vi "Variant to JSON Text.vi"(4 "LVClass Serializer":refnum<class "JSONtext LVClass Serializer.lvclass">, 5 "enable LabVIEW extensions? (T)":bool=TRUE, 6 "Pretty Print?":bool, 8 "error in (no error)":errorcluster, 10 "Variant":variant) -> (0 "error out":errorcluster, 1 "Name of data in Variant":string, 3 "<JSON>":string)   [LabVIEW 2020, in "JSONtext.lvlib"]
doc: "Converts a LabVIEW datatype (<b>Variant</b>) into a JSON value. \n\nStrings or Arrays of strings marked with a leading \"<JSON>\" tag in their name (including inside clusters) are treated as already being valid JSON. Strings not marked as <JSON> are quoted and escaped as a JSON String. Note that JSONtext.lvlib functions that produce JSON have their outputs labelled \"<JSON>\", so that they may be used as inputs to other functions.\n\nTwo types of LabVIEW Clusters are supported: either with all named elements, which are converted to JSON Objects, or all unnamed elements (or elements just named \"<JSON>\"), which are converted to a JSON Array. Handling of mixed clusters with some named and some unnamed in undefined (currently, this VI will use the first element to determine whether to convert to an Object or Array)."
uses:
  <vilib>/JDP Science/JSONtext/JSONtext.lvlib
  <vilib>/JDP Science/JSONtext/LVClass Serializer/JSONtext LVClass Serializer.lvclass
  <vilib>/Utility/Data Type/Type Definitions/Data Type.ctl
  <vilib>/JDP Science/JSONtext/support/Remove trailing zeros.vi
  <vilib>/JDP Science/JSONtext/support/quote and escape json string 2.vi
  <vilib>/JDP Science/JSONtext/Base64/base64url Encode.vi
  <vilib>/JDP Science/JSONtext/support/Format JSON Object.vi
  <vilib>/Utility/Data Type/NI_Data Type.lvlib
  <vilib>/JDP Science/JDP Science Common Utilities/JDP Utility.lvlib
  <vilib>/JDP Science/JDP Science Common Utilities/Timestamp/JDP Timestamp.lvlib
  <vilib>/JDP Science/JSONtext/support/Set Map/SetMap.lvlib
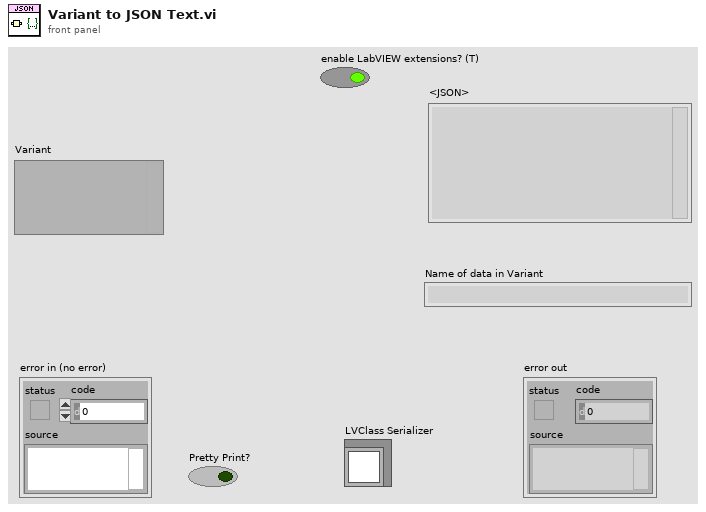
[diagram p1: front panel]
types:
  T1 = typedef "NI_Data Type.lvlib/Data Type.ctl" = enum8{"Invalid Type", "Void", "I8", "I16", "I32", "I64", "U8", "U16", "U32", "U64", "Single Float", "Double Float", "Extended Float", "Single Complex", "Double Complex", "Extended Complex", "Enum U8", "Enum U16", "Enum U32", "Enum U64", "Single Float With Unit", "Double Float With Unit", "Extended Float With Unit", "Single Complex with Unit", "Double Complex with Unit", "Extended Complex with Unit", "Boolean", "String", "Path", "Picture", "Tag", "Array", "Cluster", "Variant", "LV Variant", "Waveform", "Timestamp", "Digital Waveform", "Digital Data", "ExpressData", "Refnum", "External Data", "VI", "Poly VI", "LabVIEW Class Instance", "Fixed Point", "Set Collection", "Map Collection"}
  T2 = typedef "JSONtext.lvlib/Tag Type.ctl" = enum16{"No Tag", "<JSON>", "<JOBJ>"}
  T3 = cluster{"<JSON>attributes":string, "t0":timestamp, "dt":dbl, "Y":dbl[]}
  T4 = typedef "NI_Data Type.lvlib/Refnum Type.ctl" = enum16{"NotARefnum", "UnknownRefnum", "Generic", "Datalog", "ByteStream", "Device", "Occurence", "TCPNetConnection", "Auto", "Menu", "Imaq", "Hardware", "DataSocket", "Visa", "IVI", "UDPNetConnection", "Notifier", "Queue", "Irda", "EventReg", "DotNet", "UserEvent", "Callback", "UNUSED_EMPTY_POSITION", "BlueToothNetConnection", "LVObjApp", "LVObjVI", "LVObjUnknown", "GenericClass", "UserDefinedRefnumTag", "DataValue", "RT FIFO", "TDMS File", "PythonSessionRefnum"}
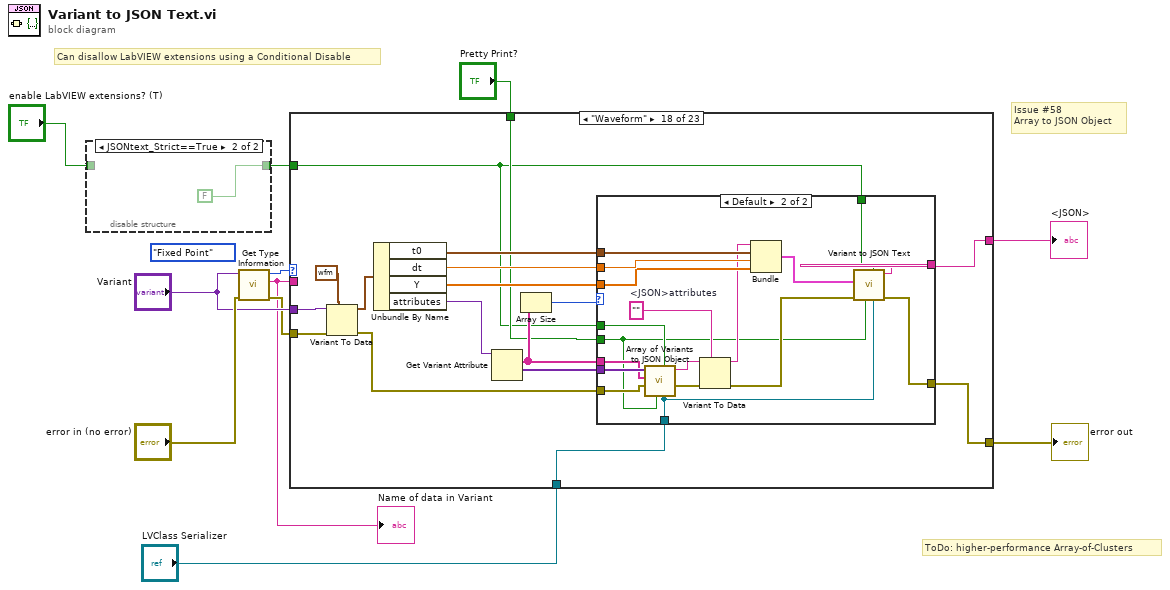
[diagram p0: block diagram]
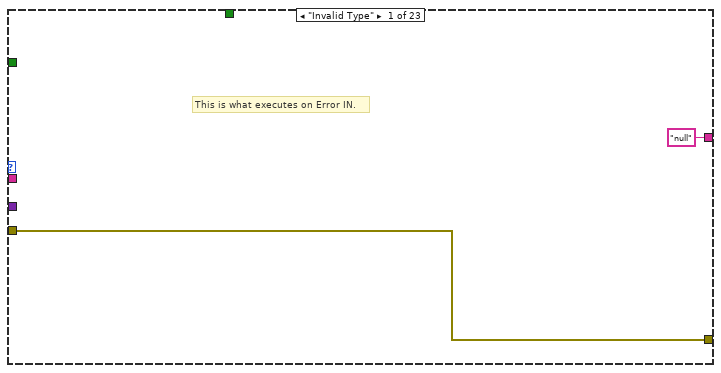
[diagram p3: hidden frame]
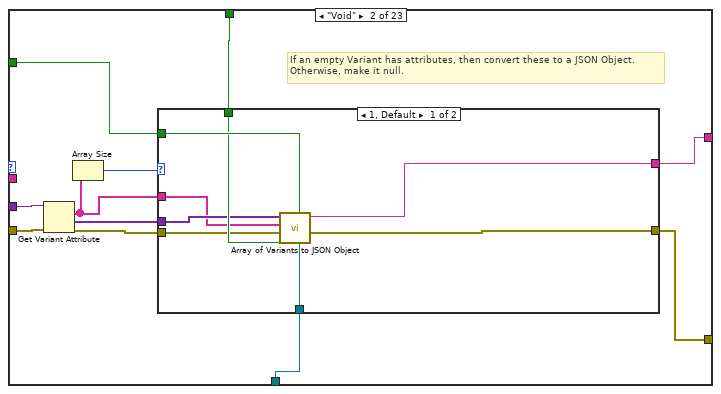
[diagram p4: hidden frame]
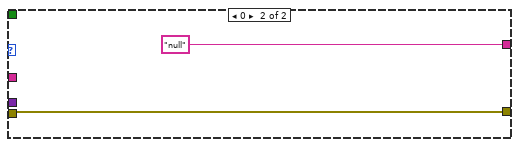
[diagram p5: hidden frame]
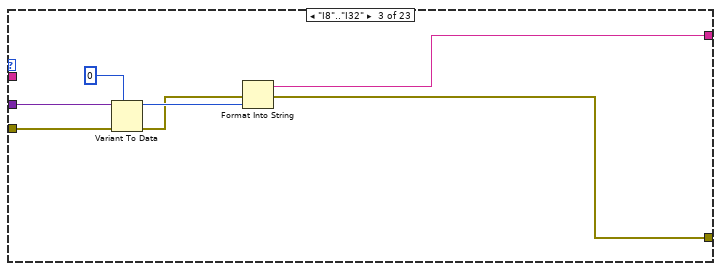
[diagram p6: hidden frame]
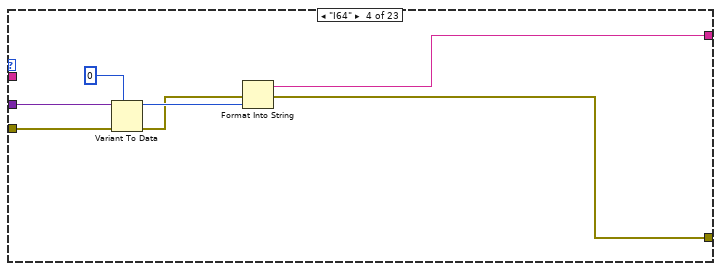
[diagram p7: hidden frame]
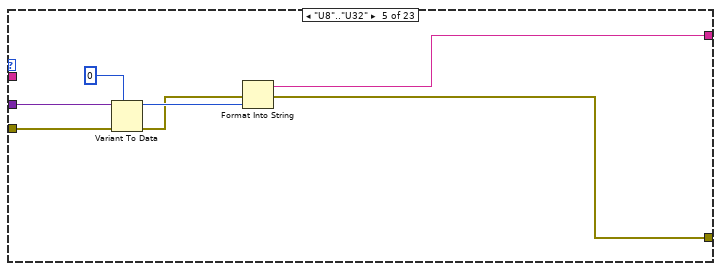
[diagram p8: hidden frame]
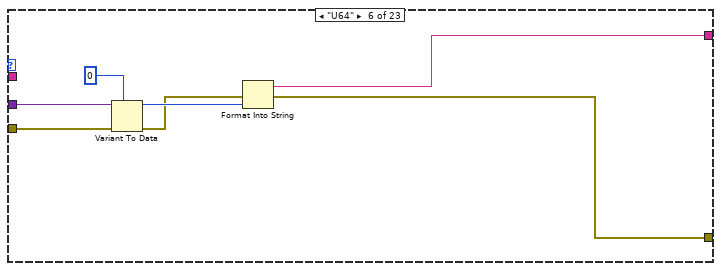
[diagram p9: hidden frame]
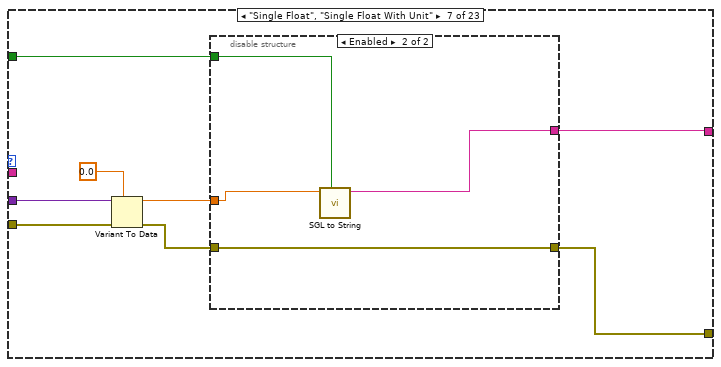
[diagram p10: hidden frame]
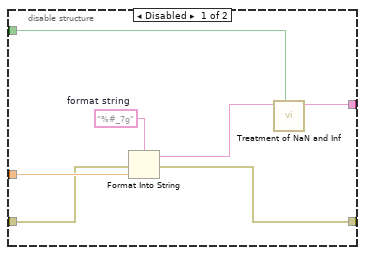
[diagram p11: hidden frame]
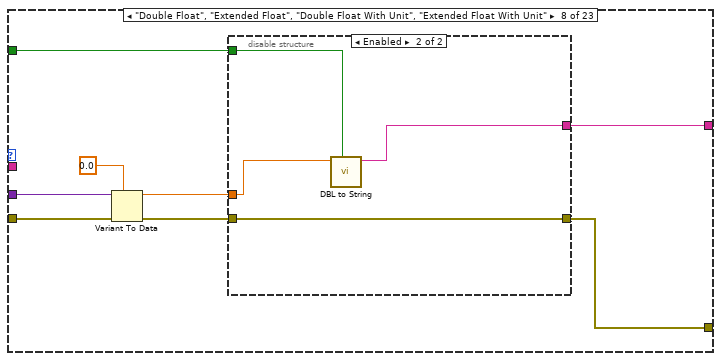
[diagram p12: hidden frame]
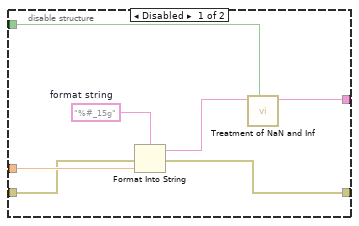
[diagram p13: hidden frame]
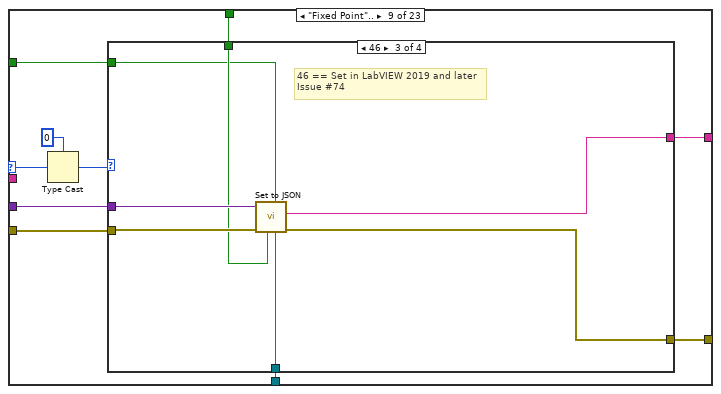
[diagram p14: hidden frame]
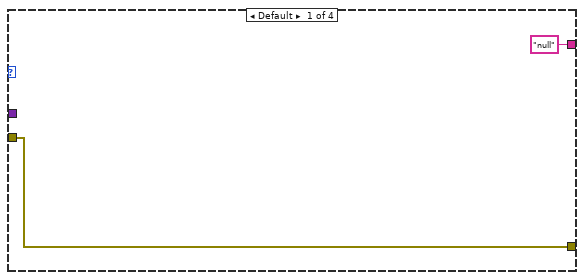
[diagram p15: hidden frame]
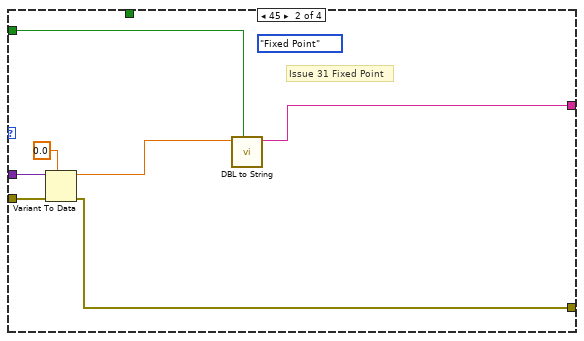
[diagram p16: hidden frame]
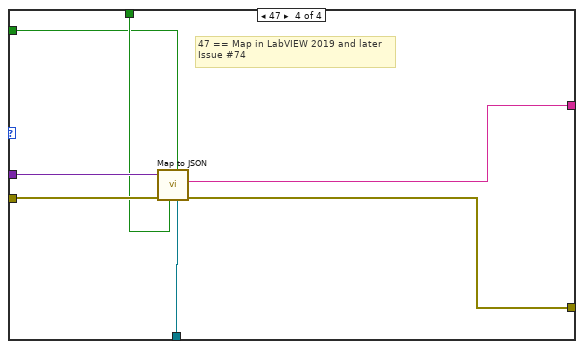
[diagram p17: hidden frame]
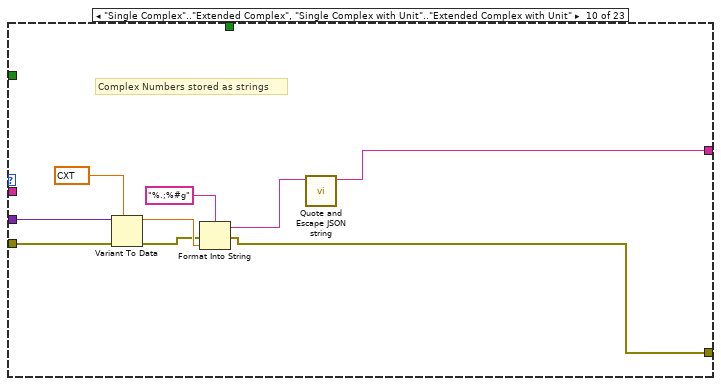
[diagram p18: hidden frame]
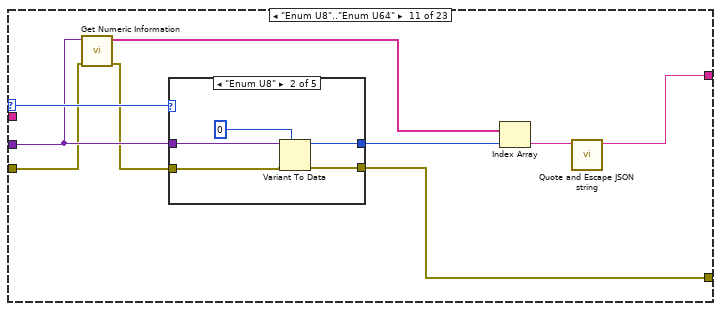
[diagram p19: hidden frame]
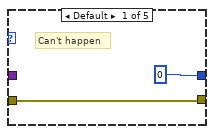
[diagram p20: hidden frame]
diagram:
  (unwired) Data_Type."Fixed Point" ("Type")
  # "ToDo: higher-performance Array-of-Clusters"
  # "Issue #58\nArray to JSON Object"
  # "Can disallow LabVIEW extensions using a Conditional Disable"
  n1 = disable-structure shown="JSONtext_Strict==True" {
    disable-tunnel: "enable LabVIEW extensions? (T)" -> [w12 _]
    disable-tunnel: [w12 FALSE ("enable LabVIEW extensions? (T)")] -> w3
    frame condition #0 (active) {
    }
    frame condition #1 {
    }
  }
  n2 = call <vilib>:"Get Type Information.vi"("error in (no error)"="error in (no error)", "variant"="Variant") -> ("error out"=w6:errorcluster, "name"=w4:string, "type"=w5:T1)  [unwired: 5 in, 2 out]
  "Name of data in Variant" <- w4
  n3 = case shown="\"Waveform\"" w5 {
    selector: w5 -> [_ _ _ _ _ _ _ _ w107 _ w152 _ _ _ _ _ _ _ _ _ _ _ _]
    tunnel: "Variant" -> [_ w25 w43 w50 w57 w64 w72 w91 w112 w144 w148 w183 w192 w204 w217 w713 w733 w754 w789 w794 w818 w830 w845]
    tunnel: [w14 w26 w37 w44 w51 w58 w67 w86 w110 w136 w147 w176 w188 w198 w218 w708 w737 w741 w783 w792 w816 w824 w842] -> w10
    tunnel: w6 -> [w14 w20 w41 w48 w55 w62 w70 w89 w111 w143 w146 w181 w187 w202 w216 w711 w732 w753 w787 w793 w817 w829 w842]
    tunnel: w4 -> [_ _ _ _ _ _ _ _ _ _ _ _ w185 _ w208 _ _ _ _ _ _ _ _]
    tunnel: ["null" ("<JSON>") w19 w39 w46 w53 w60 w66 w85 w109 w137 w150 w177 w186 w199 w210 w709 w729 w743 w784 w791 w815 w826 w843] -> w8
    tunnel: "Pretty Print?" -> [_ w18 _ _ _ _ _ _ w104 _ _ _ _ _ w211 w707 w731 w740 _ _ _ w819 _]
    tunnel: w3 -> [_ w17 _ _ _ _ w65 w84 w108 _ _ _ _ _ w209 w703 w730 w739 _ _ _ w820 _]
    tunnel: "LVClass Serializer" -> [_ w16 _ _ _ _ _ _ w103 _ _ _ _ _ w205 w702 w728 w738 _ _ _ w821 _]
    frame "Invalid Type" {
      # "This is what executes on Error IN."
    }
    frame "Void" {
      # "If an empty Variant has attributes, then convert these to a JSON Object.\nOtherwise, make it null."
      n4 = Get Variant Attribute(Variant=w25, error in=w20) -> (names=w23:string[], values=w22:variant[], error out=w21:errorcluster)  [unwired: 2 in, 1 out]
      n5 = Array Size(array=w23) -> (size(s)=w24:i32)
      n6 = case shown="1, Default" w24 {
        tunnel: [w28 w35] -> w26
        tunnel: w23 -> [w30 _]
        tunnel: w22 -> [w31 _]
        tunnel: w21 -> [w29 w35]
        tunnel: [w34 "null"] -> w19
        tunnel: w18 -> [w32 _]
        tunnel: w17 -> [w33 _]
        tunnel: w16 -> [w27 _]
        frame 1, Default {
          n7 = call <vilib>:"Array of Variants to JSON Object.vi"("LVClass Serializer"=w27, "enable LabVIEW extensions? (T)"=w33, "Pretty Print?"=w32, "error in (no error)"=w29, "Names"=w30, "Array"=w31) -> ("error out"=w28:errorcluster, "<JSON>"=w34:string)  [unwired: 4 in]
        }
        frame 0 {
        }
      }
    }
    frame "I8".."I32" {
      n8 = Variant To Data(error in=w41, type=0, Variant=w43) -> (data=w40:i32, error out=w38:errorcluster)
      n9 = Format Into String(error in=w38, w40) -> (resulting string=w39:string, error out=w37:errorcluster)  [unwired: 2 in]
    }
    frame "I64" {
      n10 = Variant To Data(error in=w48, type=i64 0, Variant=w50) -> (data=w47:i64, error out=w45:errorcluster)
      n11 = Format Into String(error in=w45, w47) -> (resulting string=w46:string, error out=w44:errorcluster)  [unwired: 2 in]
    }
    frame "U8".."U32" {
      n12 = Variant To Data(error in=w55, type=u32 0, Variant=w57) -> (data=w54:u32, error out=w52:errorcluster)
      n13 = Format Into String(error in=w52, w54) -> (resulting string=w53:string, error out=w51:errorcluster)  [unwired: 2 in]
    }
    frame "U64" {
      n14 = Variant To Data(error in=w62, type=u64 0, Variant=w64) -> (data=w61:u64, error out=w59:errorcluster)
      n15 = Format Into String(error in=w59, w61) -> (resulting string=w60:string, error out=w58:errorcluster)  [unwired: 2 in]
    }
    frame "Single Float", "Single Float With Unit" {
      n16 = Variant To Data(error in=w70, type=sgl 0.0, Variant=w72) -> (data=w69:sgl, error out=w68:errorcluster)
      n17 = disable-structure shown="Enabled" {
        disable-tunnel: w69 -> [w79 w83]
        disable-tunnel: w68 -> [w78 w81]
        disable-tunnel: [w77 w81] -> w67
        disable-tunnel: [w74 w80] -> w66
        disable-tunnel: w65 -> [w73 w82]
        frame Disabled {
          w76 = "%#_7g"  # format string
          n18 = Format Into String(format string=w76, error in=w78, w79) -> (resulting string=w75:string, error out=w77:errorcluster)  [unwired: 1 in]
          n19 = call <vilib>:"Treatment of NaN and Inf.vi"("enable LabVIEW extensions?"=w73, "Numeric Text"=w75) -> ("<JSON>"=w74:string)  [unwired: 9 in]
        }
        frame Enabled {
          n20 = call <vilib>:"SGL to String.vi"("enable LabVIEW extensions?"=w82, "SGL"=w83) -> ("SGL string"=w80:string)  [unwired: 9 in]
        }
      }
    }
    frame "Double Float", "Extended Float", "Double Float With Unit", "Extended Float With Unit" {
      n21 = Variant To Data(error in=w89, type=0.0, Variant=w91) -> (data=w88:dbl, error out=w87:errorcluster)
      n22 = disable-structure shown="Enabled" {
        disable-tunnel: w88 -> [w98 w102]
        disable-tunnel: w87 -> [w97 w99]
        disable-tunnel: [w96 w99] -> w86
        disable-tunnel: [w93 w101] -> w85
        disable-tunnel: w84 -> [w92 w100]
        frame Disabled {
          w95 = "%#_15g"  # format string
          n23 = Format Into String(format string=w95, error in=w97, w98) -> (resulting string=w94:string, error out=w96:errorcluster)  [unwired: 1 in]
          n24 = call <vilib>:"Treatment of NaN and Inf.vi"("enable LabVIEW extensions?"=w92, "Numeric Text"=w94) -> ("<JSON>"=w93:string)  [unwired: 9 in]
        }
        frame Enabled {
          n25 = call <vilib>:"DBL to String.vi"("enable LabVIEW extensions?"=w100, "DBL"=w102) -> ("DBL string"=w101:string)  [unwired: 9 in]
        }
      }
    }
    frame "Fixed Point".. {
      n26 = Type Cast(type=u8 0, x=w107) -> (*(type *) &x=w105:u8)
      n27 = case shown="46" w105 {
        tunnel: w112 -> [_ w121 w128 w135]
        tunnel: w111 -> [w113 w119 w127 w134]
        tunnel: [w113 w117 w123 w130] -> w110
        tunnel: ["null" ("<JSON>") w116 w124 w131] -> w109
        tunnel: w108 -> [_ w115 w125 w132]
        tunnel: w104 -> [_ _ w126 w133]
        tunnel: w103 -> [_ _ w122 w129]
        frame Default {
        }
        frame 45 {
          (unwired) Data_Type."Fixed Point" ("Type")
          # "Issue 31 Fixed Point"
          n28 = Variant To Data(error in=w119, type=0.0, Variant=w121) -> (data=w118:dbl, error out=w117:errorcluster)
          n29 = call <vilib>:"DBL to String.vi"("enable LabVIEW extensions?"=w115, "DBL"=w118) -> ("DBL string"=w116:string)  [unwired: 9 in]
        }
        frame 46 {
          # "46 == Set in LabVIEW 2019 and later\nIssue #74"
          n30 = call <vilib>:"Set to JSON.vi"("LVClass Serializer"=w122, "enable LabVIEW extensions?"=w125, "Pretty Print?"=w126, "error in (no error)"=w127, "Variant"=w128) -> ("error out"=w123:errorcluster, "<JSON>"=w124:string)  [unwired: 5 in]
        }
        frame 47 {
          # "47 == Map in LabVIEW 2019 and later\nIssue #74"
          n31 = call <vilib>:"Map to JSON.vi"("LVClass Serializer"=w129, "enable LabVIEW extensions?"=w132, "Pretty Print?"=w133, "error in (no error)"=w134, "Map"=w135) -> ("error out"=w130:errorcluster, "<JSON>"=w131:string)  [unwired: 5 in]
        }
      }
    }
    frame "Single Complex".."Extended Complex", "Single Complex with Unit".."Extended Complex with Unit" {
      # "Complex Numbers stored as strings"
      n32 = Variant To Data(error in=w143, type=cxt 0.0+0.0i, Variant=w144) -> (data=w141:cxt, error out=w140:errorcluster)
      n33 = Format Into String(format string="%.;%#g", error in=w140, w141) -> (resulting string=w138:string, error out=w136:errorcluster)  [unwired: 1 in]
      n34 = call <vilib>:"Quote and Escape JSON string.vi"("Plain Text"=w138) -> ("<JSON>"=w137:string)  [unwired: 10 in]
    }
    frame "Enum U8".."Enum U64" {
      n35 = call <vilib>:"Get Numeric Information.vi"("error in (no error)"=w146, "variant"=w148) -> ("error out"=w145:errorcluster, "enum names"=w149:string[])  [unwired: 6 in, 2 out]
      n36 = case shown="\"Enum U8\"" w152 {
        tunnel: [u64 0 ("U8") w159 w164 w169 w174] -> w153
        tunnel: w148 -> [_ w158 w163 w168 w173]
        tunnel: w145 -> [w154 w157 w162 w167 w172]
        tunnel: [w154 w156 w161 w166 w171] -> w147
        frame Default {
          # "Can't happen"
        }
        frame "Enum U8" {
          n37 = Variant To Data(error in=w157, type=u8 0, Variant=w158) -> (data=w159:u8, error out=w156:errorcluster)
        }
        frame "Enum U16" {
          n38 = Variant To Data(error in=w162, type=u16 0, Variant=w163) -> (data=w164:u16, error out=w161:errorcluster)
        }
        frame "Enum U32" {
          n39 = Variant To Data(error in=w167, type=u32 0, Variant=w168) -> (data=w169:u32, error out=w166:errorcluster)
        }
        frame "Enum U64" {
          w175 = u64 0  # U64
          n40 = Variant To Data(error in=w172, type=w175, Variant=w173) -> (data=w174:u64, error out=w171:errorcluster)
        }
      }
      n41 = Index Array(array=w149, index=w153) -> (element=w151:string)
      n42 = call <vilib>:"Quote and Escape JSON string.vi"("Plain Text"=w151) -> ("<JSON>"=w150:string)  [unwired: 10 in]
    }
    frame "Boolean" {
      n43 = Variant To Data(error in=w181, type=FALSE, Variant=w183) -> (data=w178:bool, error out=w176:errorcluster)
      n44 = Select(t="true", s=w178, f="false") -> (s? t:f=w177:string)
    }
    frame "String" {
      n45 = Variant To Data(error in=w187, type="", Variant=w192) -> (data=w190:string, error out=w189:errorcluster)
      n46 = call <vilib>:"Remove JSON Tag.vi"("Name"=w185) -> ("Tag"=w184:T2)  [unwired: 9 in, 1 out]
      n47 = case shown="\"No Tag\", Default" w184 {
        tunnel: w190 -> [w195 w196]
        tunnel: w189 -> [w193 w197]
        tunnel: [w193 w197] -> w188
        tunnel: [w194 w196] -> w186
        frame "No Tag", Default {
          n48 = call <vilib>:"Quote and Escape JSON string.vi"("Plain Text"=w195) -> ("<JSON>"=w194:string)  [unwired: 10 in]
        }
        frame "<JSON>" {
          # "Already JSON"
        }
      }
    }
    frame "Path" {
      n49 = Variant To Data(error in=w202, type=path "", Variant=w204) -> (data=w201:path, error out=w198:errorcluster)
      n50 = Path To String(path=w201) -> (string=w200:string)
      n51 = call <vilib>:"Quote and Escape JSON string.vi"("Plain Text"=w200) -> ("<JSON>"=w199:string)  [unwired: 10 in]
    }
    frame "Array" {
      # "Don't Pretty Print subarrays of large-dimension arrays"
      n52 = call <vilib>:"Get Array Information.vi"("error in (no error)"=w216, "variant"=w217) -> ("error out"=w214:errorcluster, "array element data type"=w213:variant, "number of dimensions"=w215:i32)  [unwired: 6 in, 1 out]
      n53 = call <vilib>:"Get Type Information.vi"("error in (no error)"=w214, "variant"=w213) -> ("error out"=w212:errorcluster, "name"=w206:string, "type"=w207:T1)  [unwired: 5 in, 2 out]
      n54 = case shown="Default" w207 {
        tunnel: [w219 w230 w630] -> w218
        tunnel: w217 -> [_ w229 w629]
        tunnel: w215 -> [_ w228 w628]
        tunnel: w212 -> [w219 w227 w627]
        tunnel: w207 -> [_ w226 _]
        tunnel: w211 -> [_ w225 w626]
        tunnel: ["null" ("JSON Object Text out") w224 w625] -> w210
        tunnel: w209 -> [_ w223 w624]
        tunnel: w208 -> [_ w222 w622]
        tunnel: w206 -> [_ _ w623]
        tunnel: w205 -> [_ w221 _]
        frame "Invalid Type" {
        }
        frame Default {
          n55 = case shown="4" w228 {
            selector: w228 -> [_ _ _ _ _ w614]
            tunnel: [w238 w392 w495 w588 w605 w620] -> w230
            tunnel: w229 -> [w239 w393 w496 w590 w607 _]
            tunnel: w227 -> [w237 w391 w494 w589 w606 w619]
            tunnel: w226 -> [w236 w390 w493 _ _ _]
            tunnel: w225 -> [w235 w389 w492 w581 w598 _]
            tunnel: [w234 w388 w491 w587 w604 "null" ("JSON Object Text out")] -> w224
            tunnel: w223 -> [w233 w387 w490 w582 w603 _]
            tunnel: w222 -> [w232 _ _ _ _ _]
            tunnel: w221 -> [w231 w386 w489 w580 w597 _]
            frame 1 {
              n56 = case shown="Default" w236 {
                tunnel: w239 -> [w247 w272 w289 w296 w317 w324 w331 w341 w354]
                tunnel: [w242 w267 w284 w291 w312 w319 w326 w334 w347] -> w238
                tunnel: w237 -> [w245 w270 w287 w294 w315 w322 w329 w339 w352]
                tunnel: w235 -> [_ _ _ _ _ _ _ w336 w349]
                tunnel: [w241 w266 w283 w290 w311 w318 w325 w337 w350] -> w234
                tunnel: w233 -> [w240 w265 _ _ _ _ _ w338 w351]
                tunnel: w232 -> [_ _ _ _ _ _ _ _ w345]
                tunnel: w231 -> [_ _ _ _ _ _ _ w332 w342]
                frame "Single Float" {
                  n57 = Variant To Data(error in=w245, type=sgl[] [], Variant=w247) -> (data=w244:sgl[], error out=w243:errorcluster)
                  n58 = disable-structure shown="Enabled" {
                    disable-tunnel: w244 -> [w252 w255 w261]
                    disable-tunnel: w243 -> [w251 w253 w263]
                    disable-tunnel: [w250 w253 w263] -> w242
                    disable-tunnel: [w249 w254 w264] -> w241
                    disable-tunnel: w240 -> [w248 _ w262]
                    frame Disabled {
                      # "Bug in 2015: Flatten to Json uses\n18 significant figures for SGL\ndata (reported to NI)."
                      n59 = Flatten To JSON(enable LabVIEW extensions? (T)=w248, anything=w252, error in (no error)=w251) -> (JSON string=w249:string, 11:w250:errorcluster)
                    }
                    frame Disabled {
                      w260 = "%_7g"  # format string
                      # "Not fast"
                      n60 = Array To Spreadsheet String(delimiter (Tab)=",", array=w255, 3:w260) -> (spreadsheet string=w258:string)
                      n61 = Concatenate Strings("[" ("string"), w258, "]" ("string")) -> (w254:string)
                    }
                    frame Enabled {
                      n62 = call <vilib>:"SGL Aray to JSON.vi"("enable LabVIEW extensions?"=w262, "SGL Array"=w261) -> ("<JSON>Array"=w264:string)  [unwired: 9 in]
                    }
                  }
                }
                frame "Double Float", "Extended Float" {
                  # "Bug in 2015: Flatten to Json uses\nonly 8 significant figures for EXT\ndata (reported to NI), so we \nconvert to DBLs"
                  n63 = Variant To Data(error in=w270, type=dbl[] [], Variant=w272) -> (data=w269:dbl[], error out=w268:errorcluster)
                  n64 = disable-structure shown="Enabled" {
                    disable-tunnel: w269 -> [w277 w281]
                    disable-tunnel: w268 -> [w276 w278]
                    disable-tunnel: [w275 w278] -> w267
                    disable-tunnel: [w274 w280] -> w266
                    disable-tunnel: w265 -> [w273 w279]
                    frame Disabled {
                      n65 = Flatten To JSON(enable LabVIEW extensions? (T)=w273, anything=w277, error in (no error)=w276) -> (JSON string=w274:string, 11:w275:errorcluster)
                    }
                    frame Enabled {
                      n66 = call <vilib>:"DBL Aray to JSON.vi"("enable LabVIEW extensions?"=w279, "DBL Array"=w281) -> ("<JSON>Array"=w280:string)  [unwired: 9 in]
                    }
                  }
                }
                frame "Path" {
                  n67 = Variant To Data(error in=w287, type=path[] [], Variant=w289) -> (data=w286:path[], error out=w285:errorcluster)
                  n68 = Path To String(path=w286) -> (string=w282:string[])
                  n69 = Flatten To JSON(anything=w282, error in (no error)=w285) -> (JSON string=w283:string, 11:w284:errorcluster)  [unwired: 1 in]
                }
                frame "I8".."I32" {
                  n70 = Variant To Data(error in=w294, type=i32[] [], Variant=w296) -> (data=w293:i32[], error out=w292:errorcluster)
                  n71 = disable-structure shown="Enabled" {
                    disable-tunnel: w293 -> [w300 w310]
                    disable-tunnel: w292 -> [w299 w301]
                    disable-tunnel: [w298 w301] -> w291
                    disable-tunnel: [w297 w306] -> w290
                    frame Enabled {
                      n72 = Flatten To JSON(anything=w300, error in (no error)=w299) -> (JSON string=w297:string, 11:w298:errorcluster)  [unwired: 1 in]
                    }
                    frame Disabled {
                      n73 = Array To Spreadsheet String(delimiter (Tab)=",", array=w310, 3:"%d" ("format string")) -> (spreadsheet string=w304:string)
                      n74 = call <vilib>:"Trim Whitespace__JDP.vi"("Remove (leading and trailing)"=enum16{"leading", "trailing", "both"}."trailing", "String in"=w304) -> ("String out"=w303:string)  [unwired: 5 in]
                      n75 = Concatenate Strings("[" ("string"), w303, "]" ("string")) -> (w306:string)
                    }
                  }
                }
                frame "I64" {
                  n76 = Variant To Data(error in=w315, type=i64[] [], Variant=w317) -> (data=w314:i64[], error out=w313:errorcluster)
                  n77 = Flatten To JSON(anything=w314, error in (no error)=w313) -> (JSON string=w311:string, 11:w312:errorcluster)  [unwired: 1 in]
                }
                frame "U8".."U32" {
                  n78 = Variant To Data(error in=w322, type=u32[] [], Variant=w324) -> (data=w321:u32[], error out=w320:errorcluster)
                  n79 = Flatten To JSON(anything=w321, error in (no error)=w320) -> (JSON string=w318:string, 11:w319:errorcluster)  [unwired: 1 in]
                }
                frame "U64" {
                  n80 = Variant To Data(error in=w329, type=u64[] [], Variant=w331) -> (data=w328:u64[], error out=w327:errorcluster)
                  n81 = Flatten To JSON(anything=w328, error in (no error)=w327) -> (JSON string=w325:string, 11:w326:errorcluster)  [unwired: 1 in]
                }
                frame Default {
                  # "Enums, etc."
                  n82 = Variant To Data(error in=w339, type=variant[] [], Variant=w341) -> (data=w333:variant[], error out=w335:errorcluster)
                  n83 = call <vilib>:"Array of Variants to JSON Array.vi"("LVClass Serializer"=w332, "enable LabVIEW extensions? (T)"=w338, "Pretty Print?"=w336, "error in (no error)"=w335, "Array of Variants"=w333) -> ("error out"=w334:errorcluster, "<JSON>"=w337:string)  [unwired: 5 in]
                }
                frame "Cluster" {
                  n84 = call <vilib>:"Remove OBJ Tag.vi"("Name"=w345) -> ("tagged as Item Name in JSON Objects"=w343:bool, "Name (tag stripped)"=w344:string)  [unwired: 9 in]
                  n85 = Variant To Data(error in=w352, type=variant[] [], Variant=w354) -> (data=w346:variant[], error out=w348:errorcluster)
                  n86 = case shown="True" w343 {
                    tunnel: w351 -> [w361 _]
                    tunnel: [w360 w364] -> w350
                    tunnel: w349 -> [w359 w363]
                    tunnel: w348 -> [w358 w369]
                    tunnel: [w357 w365] -> w347
                    tunnel: w346 -> [w356 w370]
                    tunnel: w344 -> [_ _]
                    tunnel: w342 -> [w355 w362]
                    frame False {
                      n87 = call <vilib>:"Array of Variants to JSON Array.vi"("LVClass Serializer"=w355, "enable LabVIEW extensions? (T)"=w361, "Pretty Print?"=w359, "error in (no error)"=w358, "Array of Variants"=w356) -> ("error out"=w357:errorcluster, "<JSON>"=w360:string)  [unwired: 5 in]
                    }
                    frame True {
                      n88 = for {
                        tunnel: w370 -> [w377] mode=indexing
                        shift-right: [w375] -> w366
                        shift-left: w369 -> [w380]
                        tunnel: [w374] -> w367 mode=indexing
                        tunnel: [w373] -> w368 mode=indexing
                        tunnel: w363 -> [w372]
                        tunnel: w362 -> [w371]
                        # "Issue #58 Cluster 1D Array to JOBJ"
                        n89 = Variant To Data(error in=w380, type=variant[] [], Variant=w377) -> (data=w376:variant[], error out=w379:errorcluster)
                        n90 = Index Array(array=w376) -> (element=w383:variant)  [unwired: 1 in]
                        n91 = Array Subset(array=w376, index=1) -> (w384:variant[])  [unwired: 1 in]
                        n92 = Variant To Data(error in=w379, type="", Variant=w383) -> (data=w373:string, error out=w382:errorcluster)
                        n93 = call <vilib>:"Array of Variants to JSON Object.vi"("LVClass Serializer"=w371, "Pretty Print?"=w372, "error in (no error)"=w382, "Array"=w384) -> ("error out"=w375:errorcluster, "<JSON>"=w374:string)  [unwired: 6 in]
                      }
                      n94 = call <vilib>:"Make JSON Object.vi"("Pretty Print?"=w363, "error in (no error)"=w366, "JSON Items"=w367, "Item Names"=w368) -> ("error out"=w365:errorcluster, "<JSON>"=w364:string)  [unwired: 6 in]
                    }
                  }
                }
              }
            }
            frame 2 {
              n95 = case shown="Default" w390 {
                tunnel: w393 -> [w402 w426 w448 w455 w462 w469 w481]
                tunnel: [w397 w421 w443 w450 w457 w464 w473] -> w392
                tunnel: w391 -> [w400 w424 w446 w453 w460 w467 w479]
                tunnel: w389 -> [w394 w418 _ _ _ _ w471]
                tunnel: [w396 w420 w442 w449 w456 w463 w472] -> w388
                tunnel: w387 -> [w395 w419 _ _ _ _ w476]
                tunnel: w386 -> [_ _ _ _ _ _ w470]
                frame "Single Float" {
                  n96 = Variant To Data(error in=w400, type=sgl[][] [], Variant=w402) -> (data=w399:sgl[][], error out=w398:errorcluster)
                  n97 = disable-structure shown="Enabled" {
                    disable-tunnel: w399 -> [w407 w414]
                    disable-tunnel: w398 -> [w406 w410]
                    disable-tunnel: [w405 w411] -> w397
                    disable-tunnel: [w404 w412] -> w396
                    disable-tunnel: w395 -> [w403 w409]
                    disable-tunnel: w394 -> [_ w408]
                    frame Disabled {
                      # "Bug in 2015: Flatten to Json uses\n18 significant figures for SGL\ndata (reported to NI)."
                      n98 = Flatten To JSON(enable LabVIEW extensions? (T)=w403, anything=w407, error in (no error)=w406) -> (JSON string=w404:string, 11:w405:errorcluster)
                    }
                    frame Enabled {
                      n99 = for {
                        tunnel: w414 -> [w417] mode=indexing
                        tunnel: [w416] -> w413 mode=indexing
                        tunnel: w409 -> [w415]
                        n100 = call <vilib>:"SGL Aray to JSON.vi"("enable LabVIEW extensions?"=w415, "SGL Array"=w417) -> ("<JSON>Array"=w416:string)  [unwired: 9 in]
                      }
                      n101 = call <vilib>:"Format JSON Array Text.vi"("Pretty Print?"=w408, "error in (no error)"=w410, "Array of JSON Text"=w413) -> ("error out"=w411:errorcluster, "<JSON>"=w412:string)  [unwired: 7 in]
                    }
                  }
                }
                frame "Double Float", "Extended Float" {
                  # "No easy way to support full EXT precision"
                  n102 = Variant To Data(error in=w424, type=dbl[][] [], Variant=w426) -> (data=w423:dbl[][], error out=w422:errorcluster)
                  n103 = disable-structure shown="Enabled" {
                    disable-tunnel: w423 -> [w431 w437]
                    disable-tunnel: w422 -> [w430 w436]
                    disable-tunnel: [w429 w435] -> w421
                    disable-tunnel: [w428 w434] -> w420
                    disable-tunnel: w419 -> [w427 w433]
                    disable-tunnel: w418 -> [_ w432]
                    frame Disabled {
                      # "Bug in 2015: Flatten to Json uses\n9 significant figures for EXT\ndata (reported to NI)."
                      n104 = Flatten To JSON(enable LabVIEW extensions? (T)=w427, anything=w431, error in (no error)=w430) -> (JSON string=w428:string, 11:w429:errorcluster)
                    }
                    frame Enabled {
                      n105 = for {
                        tunnel: w437 -> [w441] mode=indexing
                        tunnel: [w440] -> w438 mode=indexing
                        tunnel: w433 -> [w439]
                        n106 = call <vilib>:"DBL Aray to JSON.vi"("enable LabVIEW extensions?"=w439, "DBL Array"=w441) -> ("<JSON>Array"=w440:string)  [unwired: 9 in]
                      }
                      n107 = call <vilib>:"Format JSON Array Text.vi"("Pretty Print?"=w432, "error in (no error)"=w436, "Array of JSON Text"=w438) -> ("error out"=w435:errorcluster, "<JSON>"=w434:string)  [unwired: 7 in]
                    }
                  }
                }
                frame "I8".."I32" {
                  n108 = Variant To Data(error in=w446, type=i32[][] [], Variant=w448) -> (data=w445:i32[][], error out=w444:errorcluster)
                  n109 = Flatten To JSON(anything=w445, error in (no error)=w444) -> (JSON string=w442:string, 11:w443:errorcluster)  [unwired: 1 in]
                }
                frame "I64" {
                  n110 = Variant To Data(error in=w453, type=i64[][] [], Variant=w455) -> (data=w452:i64[][], error out=w451:errorcluster)
                  n111 = Flatten To JSON(anything=w452, error in (no error)=w451) -> (JSON string=w449:string, 11:w450:errorcluster)  [unwired: 1 in]
                }
                frame "U8".."U32" {
                  n112 = Variant To Data(error in=w460, type=u32[][] [], Variant=w462) -> (data=w459:u32[][], error out=w458:errorcluster)
                  n113 = Flatten To JSON(anything=w459, error in (no error)=w458) -> (JSON string=w456:string, 11:w457:errorcluster)  [unwired: 1 in]
                }
                frame "U64" {
                  n114 = Variant To Data(error in=w467, type=u64[][] [], Variant=w469) -> (data=w466:u64[][], error out=w465:errorcluster)
                  n115 = Flatten To JSON(anything=w466, error in (no error)=w465) -> (JSON string=w463:string, 11:w464:errorcluster)  [unwired: 1 in]
                }
                frame Default {
                  n116 = Variant To Data(error in=w479, type=variant[][] [], Variant=w481) -> (data=w474:variant[][], error out=w475:errorcluster)
                  n117 = for {
                    tunnel: w474 -> [w488] mode=indexing
                    tunnel: [w484] -> w477 mode=indexing
                    shift-right: [w487] -> w478
                    shift-left: w475 -> [w486]
                    tunnel: w476 -> [w485]
                    tunnel: w470 -> [w482]
                    n118 = call <vilib>:"Variant to JSON Text.vi"("LVClass Serializer"=w482, "enable LabVIEW extensions? (T)"=w485, "Pretty Print?"=FALSE, "error in (no error)"=w486, "Variant"=w488) -> ("error out"=w487:errorcluster, "<JSON>"=w484:string)  [unwired: 4 in, 1 out]
                  }
                  n119 = call <vilib>:"Format JSON Array Text.vi"("Pretty Print?"=w471, "error in (no error)"=w478, "Array of JSON Text"=w477) -> ("error out"=w473:errorcluster, "<JSON>"=w472:string)  [unwired: 7 in]
                }
              }
            }
            frame 3 {
              n120 = case shown="Default" w493 {
                tunnel: w496 -> [w508 w526 w540 w547 w554 w561 w573]
                tunnel: [w503 w522 w535 w542 w549 w556 w565] -> w495
                tunnel: w494 -> [w506 w524 w538 w545 w552 w559 w571]
                tunnel: w492 -> [w498 w516 _ _ _ _ w563]
                tunnel: [w502 w521 w534 w541 w548 w555 w564] -> w491
                tunnel: w490 -> [w501 w520 w533 _ _ _ w568]
                tunnel: w489 -> [w497 w515 _ _ _ _ w562]
                frame "Single Float" {
                  n121 = Variant To Data(error in=w506, type=sgl[][][] [], Variant=w508) -> (data=w505:sgl[][][], error out=w504:errorcluster)
                  n122 = for {
                    tunnel: w505 -> [w514] mode=indexing
                    tunnel: [w512] -> w500 mode=indexing
                    tunnel: w501 -> [w513]
                    shift-right: [w510] -> w499
                    shift-left: w504 -> [w511]
                    tunnel: w497 -> [w509]
                    n123 = call <vilib>:"Variant to JSON Text.vi"("LVClass Serializer"=w509, "enable LabVIEW extensions? (T)"=w513, "error in (no error)"=w511, "Variant"=w514) -> ("error out"=w510:errorcluster, "<JSON>"=w512:string)  [unwired: 5 in, 1 out]
                  }
                  n124 = call <vilib>:"Format JSON Array Text.vi"("Pretty Print?"=w498, "error in (no error)"=w499, "Array of JSON Text"=w500) -> ("error out"=w503:errorcluster, "<JSON>"=w502:string)  [unwired: 7 in]
                }
                frame "Double Float", "Extended Float" {
                  n125 = Variant To Data(error in=w524, type=dbl[][][] [], Variant=w526) -> (data=w523:dbl[][][], error out=w518:errorcluster)
                  n126 = for {
                    tunnel: w523 -> [w531] mode=indexing
                    tunnel: [w530] -> w519 mode=indexing
                    tunnel: w520 -> [w532]
                    shift-right: [w528] -> w517
                    shift-left: w518 -> [w529]
                    tunnel: w515 -> [w527]
                    n127 = call <vilib>:"Variant to JSON Text.vi"("LVClass Serializer"=w527, "enable LabVIEW extensions? (T)"=w532, "error in (no error)"=w529, "Variant"=w531) -> ("error out"=w528:errorcluster, "<JSON>"=w530:string)  [unwired: 5 in, 1 out]
                  }
                  n128 = call <vilib>:"Format JSON Array Text.vi"("Pretty Print?"=w516, "error in (no error)"=w517, "Array of JSON Text"=w519) -> ("error out"=w522:errorcluster, "<JSON>"=w521:string)  [unwired: 7 in]
                }
                frame "I8".."I32" {
                  n129 = Variant To Data(error in=w538, type=i32[][][] [], Variant=w540) -> (data=w537:i32[][][], error out=w536:errorcluster)
                  n130 = Flatten To JSON(enable LabVIEW extensions? (T)=w533, anything=w537, error in (no error)=w536) -> (JSON string=w534:string, 11:w535:errorcluster)
                }
                frame "I64" {
                  n131 = Variant To Data(error in=w545, type=i64[][][] [], Variant=w547) -> (data=w544:i64[][][], error out=w543:errorcluster)
                  n132 = Flatten To JSON(anything=w544, error in (no error)=w543) -> (JSON string=w541:string, 11:w542:errorcluster)  [unwired: 1 in]
                }
                frame "U8".."U32" {
                  n133 = Variant To Data(error in=w552, type=u32[][][] [], Variant=w554) -> (data=w551:u32[][][], error out=w550:errorcluster)
                  n134 = Flatten To JSON(anything=w551, error in (no error)=w550) -> (JSON string=w548:string, 11:w549:errorcluster)  [unwired: 1 in]
                }
                frame "U64" {
                  n135 = Variant To Data(error in=w559, type=u64[][][] [], Variant=w561) -> (data=w558:u64[][][], error out=w557:errorcluster)
                  n136 = Flatten To JSON(anything=w558, error in (no error)=w557) -> (JSON string=w555:string, 11:w556:errorcluster)  [unwired: 1 in]
                }
                frame Default {
                  n137 = Variant To Data(error in=w571, type=variant[][][] [], Variant=w573) -> (data=w566:variant[][][], error out=w567:errorcluster)
                  n138 = for {
                    tunnel: w566 -> [w579] mode=indexing
                    tunnel: [w575] -> w569 mode=indexing
                    shift-right: [w578] -> w570
                    shift-left: w567 -> [w577]
                    tunnel: w568 -> [w576]
                    tunnel: w562 -> [w574]
                    n139 = call <vilib>:"Variant to JSON Text.vi"("LVClass Serializer"=w574, "enable LabVIEW extensions? (T)"=w576, "error in (no error)"=w577, "Variant"=w579) -> ("error out"=w578:errorcluster, "<JSON>"=w575:string)  [unwired: 5 in, 1 out]
                  }
                  n140 = call <vilib>:"Format JSON Array Text.vi"("Pretty Print?"=w563, "error in (no error)"=w570, "Array of JSON Text"=w569) -> ("error out"=w565:errorcluster, "<JSON>"=w564:string)  [unwired: 7 in]
                }
              }
            }
            frame 4 {
              n141 = Variant To Data(error in=w589, type=variant[][][][] [], Variant=w590) -> (data=w585:variant[][][][], error out=w584:errorcluster)
              n142 = for {
                tunnel: w585 -> [w596] mode=indexing
                shift-right: [w594] -> w588
                shift-left: w584 -> [w595]
                tunnel: [w592] -> w583 mode=indexing
                tunnel: w582 -> [w593]
                tunnel: w580 -> [w591]
                n143 = call <vilib>:"Variant to JSON Text.vi"("LVClass Serializer"=w591, "enable LabVIEW extensions? (T)"=w593, "error in (no error)"=w595, "Variant"=w596) -> ("error out"=w594:errorcluster, "<JSON>"=w592:string)  [unwired: 5 in, 1 out]
              }
              n144 = call <vilib>:"Format JSON Array Text.vi"("Pretty Print?"=w581, "Array of JSON Text"=w583) -> ("<JSON>"=w587:string)  [unwired: 8 in, 1 out]
            }
            frame 5 {
              n145 = Variant To Data(error in=w606, type=variant[][][][][] [], Variant=w607) -> (data=w601:variant[][][][][], error out=w600:errorcluster)
              n146 = for {
                tunnel: w601 -> [w613] mode=indexing
                shift-right: [w611] -> w605
                shift-left: w600 -> [w612]
                tunnel: [w609] -> w599 mode=indexing
                tunnel: w603 -> [w610]
                tunnel: w597 -> [w608]
                n147 = call <vilib>:"Variant to JSON Text.vi"("LVClass Serializer"=w608, "enable LabVIEW extensions? (T)"=w610, "error in (no error)"=w612, "Variant"=w613) -> ("error out"=w611:errorcluster, "<JSON>"=w609:string)  [unwired: 5 in, 1 out]
              }
              n148 = call <vilib>:"Format JSON Array Text.vi"("Pretty Print?"=w598, "Array of JSON Text"=w599) -> ("<JSON>"=w604:string)  [unwired: 8 in, 1 out]
            }
            frame Default {
              n149 = Format Into String(format string="Can't support array of dim=%d", w614) -> (resulting string=w617:string)  [unwired: 2 in, 1 out]
              n150 = call <vilib>:"Error Cluster From Error Code.vi"("error in (no error)"=w619, "error message (\"\")"=w617, "error code (0)"=402843) -> ("error out"=w620:errorcluster)  [unwired: 6 in]
            }
          }
        }
        frame "String" {
          n151 = call <vilib>:"JSON Tags on Array.vi"("Array Name"=w622, "Element Name"=w623) -> ("Tag"=w621:T2)  [unwired: 9 in]
          n152 = case shown="\"No Tag\", Default" w621 {
            tunnel: [w634 w673] -> w630
            tunnel: w629 -> [w637 w672]
            tunnel: w628 -> [w631 w671]
            tunnel: w627 -> [w636 w670]
            tunnel: w626 -> [w632 w669]
            tunnel: [w635 w668] -> w625
            tunnel: w624 -> [w633 w667]
            frame "<JSON>" {
              # "JSON text --> can't use LV primative"
              n153 = case shown="0, Default" w631 {
                selector: w631 -> [w639 _ _]
                tunnel: w637 -> [_ w651 w661]
                tunnel: w636 -> [w640 w650 w660]
                tunnel: ["null" ("<JSON>") w648 w653] -> w635
                tunnel: [w638 w649 w655] -> w634
                tunnel: w633 -> [_ _ _]
                tunnel: w632 -> [_ w647 w654]
                frame 0, Default {
                  n154 = Format Into String(format string="Can't support array of dim=%d", w639) -> (resulting string=w642:string)  [unwired: 2 in, 1 out]
                  n155 = call <vilib>:"Error Cluster From Error Code.vi"("error in (no error)"=w640, "error message (\"\")"=w642, "error code (0)"=402843) -> ("error out"=w638:errorcluster)  [unwired: 6 in]
                }
                frame 1 {
                  n156 = Variant To Data(error in=w650, type=string[] [], Variant=w651) -> (data=w645:string[], error out=w646:errorcluster)
                  n157 = call <vilib>:"Format JSON Array Text.vi"("Pretty Print?"=w647, "error in (no error)"=w646, "Array of JSON Text"=w645) -> ("error out"=w649:errorcluster, "<JSON>"=w648:string)  [unwired: 7 in]
                }
                frame 2 {
                  n158 = Variant To Data(error in=w660, type=string[][] [], Variant=w661) -> (data=w658:string[][], error out=w659:errorcluster)
                  n159 = for {
                    tunnel: [w665] -> w657 mode=indexing
                    tunnel: w658 -> [w663] mode=indexing
                    shift-right: [w666] -> w656
                    shift-left: w659 -> [w664]
                    n160 = call <vilib>:"Format JSON Array Text.vi"("error in (no error)"=w664, "Array of JSON Text"=w663) -> ("error out"=w666:errorcluster, "<JSON>"=w665:string)  [unwired: 8 in]
                  }
                  n161 = call <vilib>:"Format JSON Array Text.vi"("Pretty Print?"=w654, "error in (no error)"=w656, "Array of JSON Text"=w657) -> ("error out"=w655:errorcluster, "<JSON>"=w653:string)  [unwired: 7 in]
                }
              }
            }
            frame "No Tag", Default {
              # "Note: LV JSON primative does work with zero bytes."
              n162 = case shown="1" w671 {
                selector: w671 -> [_ _ _ w695]
                tunnel: [w679 w686 w693 w701] -> w673
                tunnel: w672 -> [w680 w687 w694 _]
                tunnel: w670 -> [w678 w685 w692 w700]
                tunnel: w669 -> [_ _ _ _]
                tunnel: [w677 w684 w691 "null" ("JSON Object Text out")] -> w668
                tunnel: w667 -> [_ _ _ _]
                frame 1 {
                  n163 = Variant To Data(error in=w678, type=string[] [], Variant=w680) -> (data=w675:string[], error out=w674:errorcluster)
                  n164 = Flatten To JSON(anything=w675, error in (no error)=w674) -> (JSON string=w677:string, 11:w679:errorcluster)  [unwired: 1 in]
                }
                frame 2 {
                  n165 = Variant To Data(error in=w685, type=string[][] [], Variant=w687) -> (data=w682:string[][], error out=w681:errorcluster)
                  n166 = Flatten To JSON(anything=w682, error in (no error)=w681) -> (JSON string=w684:string, 11:w686:errorcluster)  [unwired: 1 in]
                }
                frame 3 {
                  n167 = Variant To Data(error in=w692, type=string[][][] [], Variant=w694) -> (data=w689:string[][][], error out=w688:errorcluster)
                  n168 = Flatten To JSON(anything=w689, error in (no error)=w688) -> (JSON string=w691:string, 11:w693:errorcluster)  [unwired: 1 in]
                }
                frame Default {
                  n169 = Format Into String(format string="Can't support array of dim=%d", w695) -> (resulting string=w698:string)  [unwired: 2 in, 1 out]
                  n170 = call <vilib>:"Error Cluster From Error Code.vi"("error in (no error)"=w700, "error message (\"\")"=w698, "error code (0)"=402843) -> ("error out"=w701:errorcluster)  [unwired: 6 in]
                }
              }
            }
          }
        }
      }
    }
    frame "Cluster" {
      # "Cluster of unnamed (possibly with <JSON>tags) to JSON Array?"
      n171 = Variant To Data(error in=w711, type=variant[] [], Variant=w713) -> (data=w706:variant[], error out=w712:errorcluster)
      n172 = Index Array(array=w706) -> (element=w705:variant)  [unwired: 1 in]
      n173 = call <vilib>:"Get Type Information.vi"("variant"=w705) -> ("name"=w704:string)  [unwired: 6 in, 4 out]
      n174 = case shown="Default" w704 {
        tunnel: w712 -> [w717 w723]
        tunnel: [w715 w727] -> w709
        tunnel: [w716 w722] -> w708
        tunnel: w707 -> [w719 w725]
        tunnel: w706 -> [w718 w724]
        tunnel: w703 -> [w720 w726]
        tunnel: w702 -> [w714 w721]
        frame Default {
          n175 = call <vilib>:"Array of Variants to JSON Object.vi"("LVClass Serializer"=w714, "enable LabVIEW extensions? (T)"=w720, "Pretty Print?"=w719, "error in (no error)"=w717, "Array"=w718) -> ("error out"=w716:errorcluster, "<JSON>"=w715:string)  [unwired: 5 in]
        }
        frame "", "<JSON>" {
          n176 = call <vilib>:"Array of Variants to JSON Array.vi"("LVClass Serializer"=w721, "enable LabVIEW extensions? (T)"=w726, "Pretty Print?"=w725, "error in (no error)"=w723, "Array of Variants"=w724) -> ("error out"=w722:errorcluster, "<JSON>"=w727:string)  [unwired: 5 in]
        }
      }
    }
    frame "Variant", "LV Variant" {
      n177 = Variant To Data(error in=w732, type=variant, Variant=w733) -> (data=w736:variant, error out=w735:errorcluster)
      n178 = call <vilib>:"Variant to JSON Text.vi"("LVClass Serializer"=w728, "enable LabVIEW extensions? (T)"=w730, "Pretty Print?"=w731, "error in (no error)"=w735, "Variant"=w736) -> ("error out"=w737:errorcluster, "<JSON>"=w729:string)  [unwired: 4 in, 1 out]
    }
    frame "Waveform" {
      n179 = Variant To Data(error in=w753, type=waveform(dbl) {"t0"=timestamp(0 s since 1904-01-01), "dt"=1.0, "Y"=[]} ("waveform"), Variant=w754) -> (data=w751:waveform(dbl), error out=w742:errorcluster)
      n180 = Unbundle By Name(w751) -> ("t0"=w750:timestamp, "dt"=w749:dbl, "Y"=w748:dbl[], "attributes"=w747:variant)
      n181 = Get Variant Attribute(Variant=w747) -> (names=w744:string[], values=w745:variant[])  [unwired: 3 in, 2 out]
      n182 = Array Size(array=w744) -> (size(s)=w746:i32)
      n183 = case shown="Default" w746 {
        tunnel: w750 -> [w764 w782]
        tunnel: w749 -> [w763 w781]
        tunnel: w748 -> [w762 w780]
        tunnel: [w756 w772] -> w743
        tunnel: w745 -> [_ w770]
        tunnel: w744 -> [_ w767]
        tunnel: w740 -> [w757 w765]
        tunnel: w742 -> [w760 w769]
        tunnel: [w759 w776] -> w741
        tunnel: w739 -> [w758 w773]
        tunnel: w739 -> [_ w771]
        tunnel: w738 -> [w755 w766]
        frame 0 {
          # "No Attributes"
          n184 = Bundle("t0"=w764, "dt"=w763, "Y"=w762) -> (w761:cluster{"t0":timestamp, "dt":dbl, "Y":dbl[]})  [unwired: 1 in]
          n185 = call <vilib>:"Variant to JSON Text.vi"("LVClass Serializer"=w755, "enable LabVIEW extensions? (T)"=w758, "Pretty Print?"=w757, "error in (no error)"=w760, "Variant"=w761) -> ("error out"=w759:errorcluster, "<JSON>"=w756:string)  [unwired: 4 in, 1 out]
        }
        frame Default {
          w778 = ""  # <JSON>attributes
          n186 = call <vilib>:"Array of Variants to JSON Object.vi"("LVClass Serializer"=w766, "enable LabVIEW extensions? (T)"=w771, "Pretty Print?"=w765, "error in (no error)"=w769, "Names"=w767, "Array"=w770) -> ("error out"=w768:errorcluster, "<JSON>"=w779:string)  [unwired: 4 in]
          n187 = Variant To Data(error in=w768, type=w778, Variant=w779) -> (data=w774:string, error out=w775:errorcluster)
          n188 = Bundle("<JSON>attributes"=w774, "t0"=w782, "dt"=w781, "Y"=w780) -> (w777:T3)  [unwired: 1 in]
          n189 = call <vilib>:"Variant to JSON Text.vi"("LVClass Serializer"=w766, "enable LabVIEW extensions? (T)"=w773, "Pretty Print?"=w765, "error in (no error)"=w775, "Variant"=w777) -> ("error out"=w776:errorcluster, "<JSON>"=w772:string)  [unwired: 4 in, 1 out]
        }
      }
    }
    frame "Timestamp" {
      n190 = Variant To Data(error in=w787, type=timestamp(0 s since 1904-01-01), Variant=w789) -> (data=w786:timestamp, error out=w783:errorcluster)
      n191 = call <vilib>:"Timestamp to Text.vi"("Time Stamp"=w786) -> ("Timestamp (RFC3339)"=w785:string)  [unwired: 9 in, 1 out]
      n192 = call <vilib>:"Quote and Escape JSON string.vi"("Plain Text"=w785) -> ("<JSON>"=w784:string)  [unwired: 10 in]
    }
    frame "Refnum" {
      n193 = call <vilib>:"Get Refnum Information.vi"("error in (no error)"=w793, "variant"=w794) -> ("error out"=w796:errorcluster, "reference type"=w795:T4)  [unwired: 6 in, 2 out]
      n194 = case shown="Default" w795 {
        selector: w795 -> [_ _ w807]
        tunnel: ["null" w800 w808] -> w790
        tunnel: w796 -> [w797 w802 w810]
        tunnel: [w797 w799 w809] -> w792
        tunnel: w794 -> [_ w803 w812]
        frame "NotARefnum", "UnknownRefnum" {
        }
        frame "Visa", "IVI", "UserDefinedRefnumTag" {
          n195 = Variant To Data(error in=w802, type="", Variant=w803) -> (data=w800:string, error out=w799:errorcluster)
        }
        frame Default {
          # "Store refnums in Hex (use case: routing back replies)"
          n196 = Variant To Flattened String(Variant=w812) -> (data string=w811:string)  [unwired: 1 out]
          n197 = Type Cast(type=u32 0, x=w811) -> (*(type *) &x=w804:u32)
          n198 = Format Into String(format string="%s->%x", error in=w810, w807, w804) -> (resulting string=w808:string, error out=w809:errorcluster)  [unwired: 1 in]
        }
      }
      n199 = call <vilib>:"Quote and Escape JSON string.vi"("Plain Text"=w790) -> ("<JSON>"=w791:string)  [unwired: 10 in]
    }
    frame "Tag" {
      # "Issue 37, handle DAQmx Tags"
      n200 = Variant To Data(error in=w817, type="", Variant=w818) -> (data=w814:string, error out=w816:errorcluster)
      n201 = call <vilib>:"Quote and Escape JSON string.vi"("Plain Text"=w814) -> ("<JSON>"=w815:string)  [unwired: 10 in]
    }
    frame "LabVIEW Class Instance" {
      w823 = refnum<class "JSONtext LVClass Serializer.lvclass"> refnum  # Default Flattening
      n202 = Variant To Data(error in=w829, type=refnum<class> refnum ("LabVIEW Object"), Variant=w830) -> (data=w827:refnum<class>, error out=w825:errorcluster)
      n203 = Not Equal?(x=w821, y=w823) -> (x != y?=w822:bool)
      n204 = case shown="True" w822 {
        tunnel: w827 -> [w834 w838]
        tunnel: [w833 w839] -> w826
        tunnel: w825 -> [w832 w841]
        tunnel: [w831 w840] -> w824
        tunnel: w821 -> [_ w837]
        tunnel: w820 -> [_ w836]
        tunnel: w819 -> [_ w835]
        frame False {
          n205 = call <vilib>:"LVObject to JSON.vi"("error in (no error)"=w832, "LabVIEW Object in"=w834) -> ("error out"=w831:errorcluster, "<JSON>"=w833:string)  [unwired: 8 in]
        }
        frame True {
          # "Issue #56 Way of providing alternate format\nof LVObjects"
          n206 = call-dynamic <vilib>:"LVObject to JSON.vi"("enable LabVIEW extensions? (T)"=w836, "Pretty Print?"=w835, "JSONtext LVClass Serializer in"=w837, "error in (no error)"=w841, "Object"=w838) -> ("error out"=w840:errorcluster, "<JSON>Object"=w839:string)  [unwired: 5 in]
        }
      }
    }
    frame Default {
      # "For lack of a better thing to do,\nflatten to string."
      n207 = Variant To Flattened String(Variant=w845) -> (data string=w844:string)  [unwired: 1 out]
      n208 = call <vilib>:"Quote and Escape JSON string.vi"("Plain Text"=w844) -> ("<JSON>"=w843:string)  [unwired: 10 in]
    }
  }
  "error out" <- w10
  "<JSON>" <- w8
